vi "Get Domain.vi"(7 "target Domain":refnum<class "NI_Domain.lvclass">, 8 "error in (no error)":errorcluster, 11 "PDE in":refnum<class "NI_PDE.lvclass">) -> (0 "error out":errorcluster, 2 "domain":variant, 3 "PDE out":refnum<class "NI_PDE.lvclass">)   [LabVIEW 2020, in "NI_PDE.lvlib" / "NI_PDE.lvclass"]
uses:
  <vilib>/gmath/pde.llb/PDEClass/NI_PDE.lvclass
  <vilib>/gmath/pde.llb/DomainClass/NI_Domain.lvclass
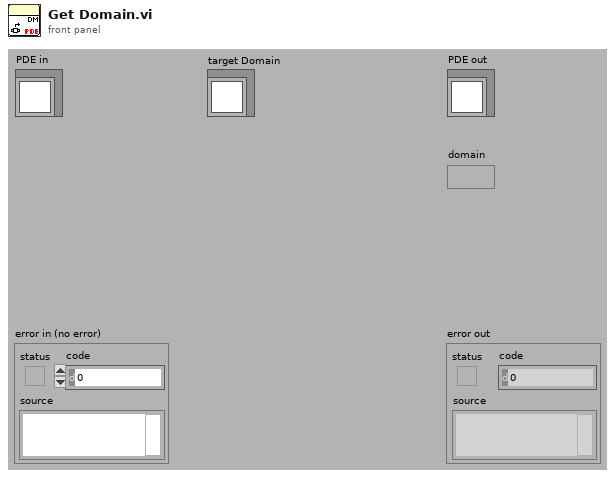
[diagram p1: front panel]
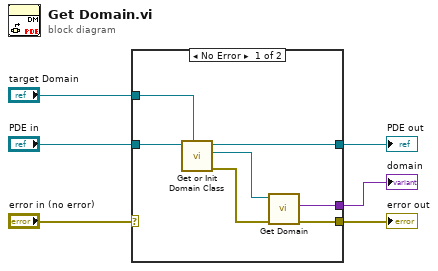
[diagram p0: block diagram]
diagram:
  n1 = case shown="No Error" "error in (no error)" {
    selector: "error in (no error)" -> [_ w14]
    tunnel: [w9 w14] -> w6
    tunnel: "PDE in" -> [w13 w15]
    tunnel: [w12 w15] -> w4
    tunnel: "target Domain" -> [w11 _]
    tunnel: [w7 _] -> w1
    frame No Error {
      n2 = call <vilib>:"Get or Init Domain Class.vi"("target Domain"=w11, "PDE out"=w13) -> ("error out"=w10:errorcluster, "Domain out"=w8:refnum<class "NI_Domain.lvclass">, "PDE in"=w12:refnum<class "NI_PDE.lvclass">)  [unwired: 1 in, 6 out]
      n3 = call-dynamic "Get Domain.vi"("error in (no error)"=w10, "Domain in"=w8) -> ("error out"=w9:errorcluster, "domain"=w7:variant)  [unwired: 8 out]
    }
    frame Error {
    }
  }
  "error out" <- w6
  "PDE out" <- w4
  "domain" <- w1
